vi "Customizing Dial.vi"() -> ()   [LabVIEW 2018]
panel:
  in  "Dial 3":i8(knob) scale=0.0..2.0
  in  "Dial 2":i8(knob) scale=0.0..2.0
  in  "Dial 1":i8(knob) scale=0.0..10.0
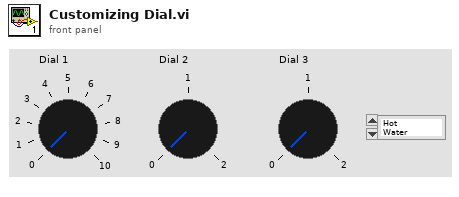
[diagram p1: front panel]
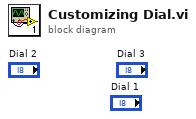
[diagram p0: block diagram]
diagram:
